vi "solar_excel Worksheet Write (Range).vi"(8 "error in (no error)":errorcluster, 9 "Cells":string[][](array[string]), 10 "Start (1,1 = 'A1')":cluster{"Row":u32, "Column":u32}, 11 "Excel Worksheet in":T1) -> (0 "error out":errorcluster, 3 "Excel Worksheet out":T1)   [LabVIEW 2018]
doc: "This writes <b>Cells</b> to a Worksheet specified by the <b>Start</b> cell range."
uses:
  solar_excel_ctl Worksheet.ctl
  solar_excel_ctl TSV.ctl
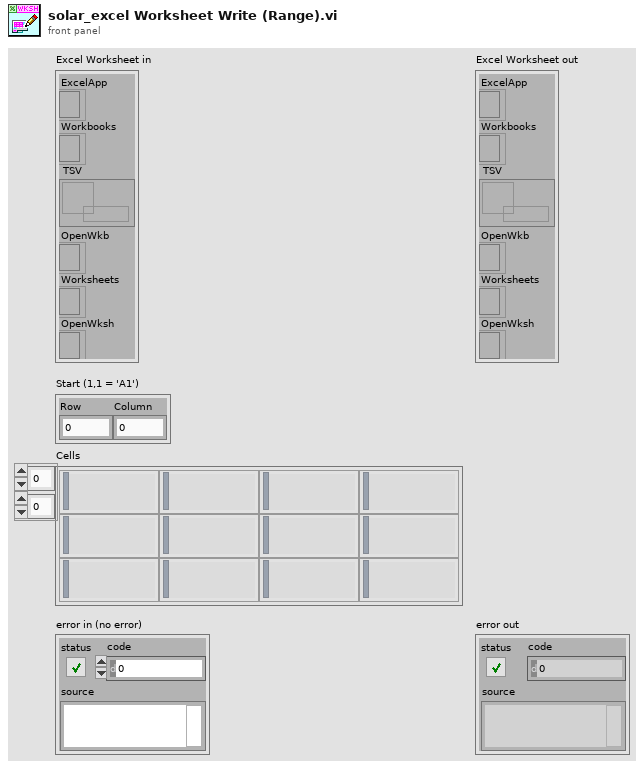
[diagram p1: front panel]
types:
  T1 = typedef "solar_excel_ctl Worksheet.ctl" = cluster{"ExcelApp":refnum<k7>, "Workbooks":refnum<k7>, "TSV":refnum<queue>, "OpenWkb":refnum<k7>, "Worksheets":refnum<k7>, "OpenWksh":refnum<k7>}
  T2 = typedef "solar_excel_ctl TSV.ctl" = cluster{"Path":path, "Dirty":bool, "ActiveSheet":u8, "Worksheets":string[], "Worksheet Cells":cluster{"Cells":string[][]}[]}
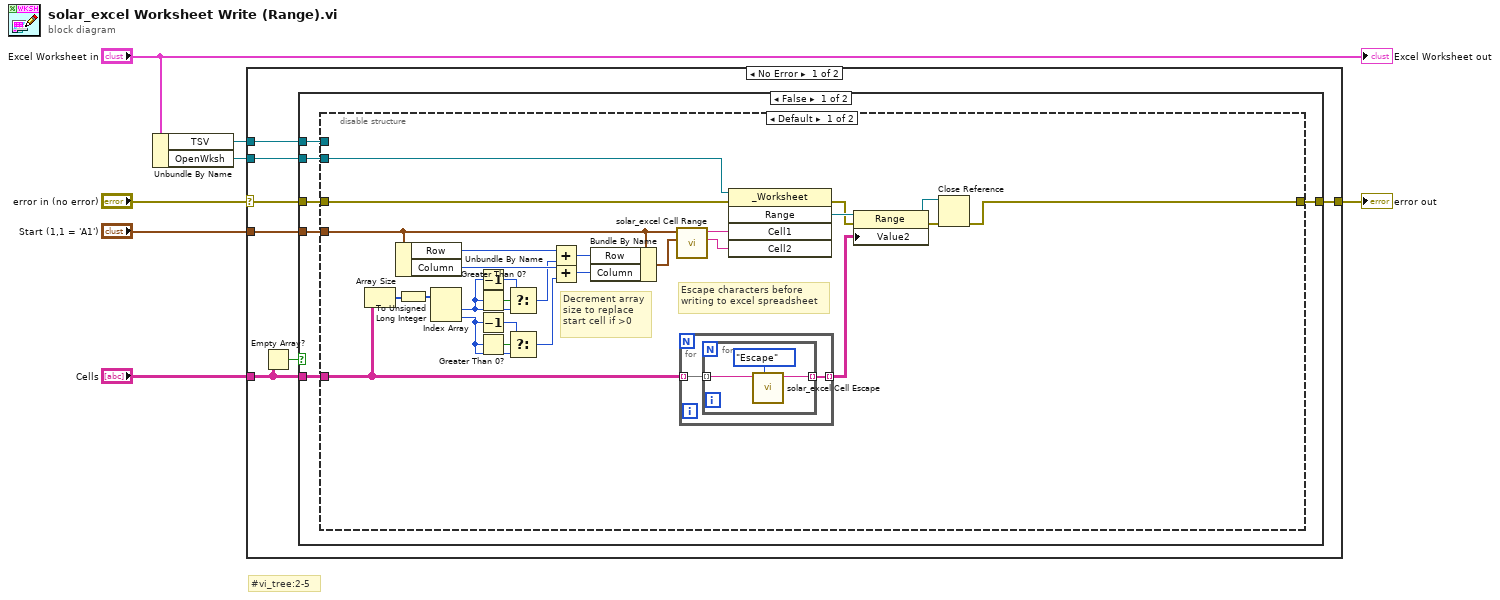
[diagram p0: block diagram]
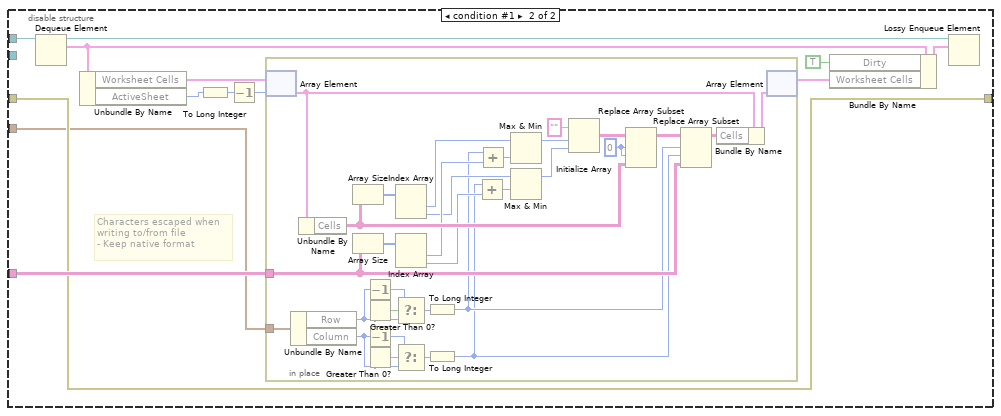
[diagram p2: hidden frame]
diagram:
  # "#vi_tree:2-5"
  n1 = Unbundle By Name("Excel Worksheet in") -> ("TSV"=w1:refnum<queue>, "OpenWksh"=w5:refnum<k7>)
  n2 = case shown="No Error" "error in (no error)" {
    selector: "error in (no error)" -> [w14 w97]
    tunnel: [w12 w97] -> w7
    tunnel: w5 -> [w13 _]
    tunnel: "Start (1,1 = 'A1')" -> [w11 _]
    tunnel: "Cells" -> [w10 _]
    tunnel: w1 -> [w8 _]
    frame No Error {
      n3 = Empty Array?(array=w10) -> (empty?=w9:bool)
      n4 = case shown="False" w9 {
        tunnel: w14 -> [w20 w96]
        tunnel: w13 -> [w19 _]
        tunnel: [w18 w96] -> w12
        tunnel: w10 -> [w17 _]
        tunnel: w11 -> [w16 _]
        tunnel: w8 -> [w15 _]
        frame False {
          n5 = disable-structure shown="Default" {
            disable-tunnel: w20 -> [w47 w54]
            disable-tunnel: w19 -> [w46 _]
            disable-tunnel: [w39 w54] -> w18
            disable-tunnel: w17 -> [w22 w55]
            disable-tunnel: w16 -> [w38 w53]
            disable-tunnel: w15 -> [_ w65]
            frame condition #0 (active) {
              # "Escape characters before\nwriting to excel spreadsheet"
              # "Decrement array\nsize to replace\nstart cell if >0"
              n6 = Array Size(array=w22) -> (size(s)=w36:i32[])
              n7 = Unbundle By Name(w38) -> ("Row"=w35:u32, "Column"=w32:u32)
              n8 = To Unsigned Long Integer(number=w36) -> (unsigned 32bit integer=w33:u32[])
              n9 = Index Array(array=w33) -> (element #1=w24:u32, element #2=w29:u32)  [unwired: 2 in]
              n10 = Decrement(x=w24) -> (x-1=w26:u32)
              n11 = Greater Than 0?(x=w24) -> (x > 0?=w25:bool)
              n12 = Decrement(x=w29) -> (x-1=w28:u32)
              n13 = Greater Than 0?(x=w29) -> (x > 0?=w30:bool)
              n14 = Select(t=w26, s=w25, f=w24) -> (s? t:f=w23:u32)
              n15 = Select(t=w28, s=w30, f=w29) -> (s? t:f=w27:u32)
              n16 = Add(x=w35, y=w23) -> (x+y=w34:u32)
              n17 = Add(x=w32, y=w27) -> (x+y=w31:u32)
              n18 = Bundle By Name(cluster=w38, "Row"=w34, "Column"=w31) -> (w37:cluster{"Row":u32, "Column":u32})
              n19 = call "solar_excel Cell Range.vi"("End (1,1 = 'A1')"=w37, "Start (1,1 = 'A1')"=w38) -> ("End Cell"=w40:string, "Start Cell"=w41:string)  [unwired: 7 in, 1 out]
              n20 = for {
                tunnel: w22 -> [w49] mode=indexing
                tunnel: [w48] -> w21 mode=indexing
                n21 = for {
                  tunnel: w49 -> [w52] mode=indexing
                  tunnel: [w50] -> w48 mode=indexing
                  n22 = call "solar_excel Cell Escape.vi"("Action (Escape)"=enum8{"Escape", "Unescape"}."Escape", "String in"=w52) -> ("String out"=w50:string)  [unwired: 9 in]
                }
              }
              n23 = invoke class="_Worksheet" method="Range"(reference=w46, error in=w47, "Cell1"=w41, "Cell2"=w40) -> (error out=w44:errorcluster, "Range"=w45:refnum<k7>)  [unwired: 1 in, 3 out]
              n24 = property class="Range"(reference=w45, error in=w44, "Value2"=w21) -> (reference out=w42:refnum<k7>, error out=w43:errorcluster)
              n25 = Close Reference(reference=w42, error in (no error)=w43) -> (error out=w39:errorcluster)
            }
            frame condition #1 {
              # "Characters escaped when\nwriting to/from file\n- Keep native format"
              n26 = Dequeue Element(queue=w65) -> (queue out=w64:refnum<queue>, element=w63:T2)  [unwired: 2 in, 2 out]
              n27 = Unbundle By Name(w63) -> ("Worksheet Cells"=w62:cluster{"Cells":string[][]}[], "ActiveSheet"=w61:u8)
              n28 = To Long Integer(number=w61) -> (32bit integer=w60:i32)
              n29 = Decrement(x=w60) -> (x-1=w59:i32)
              n30 = in-place {
                in-place-border: w55 -> [w91]
                in-place-border: w53 -> [w90]
                w77 = 0 ("disabled index (col)")
                n31 = in-place-array #1(w62, w59) -> (w95:cluster{"Cells":string[][]})
                n32 = Unbundle By Name(w90) -> ("Row"=w73:u32, "Column"=w70:u32)
                n33 = Unbundle By Name(w95) -> ("Cells"=w92:string[][])
                n34 = Array Size(array=w92) -> (size(s)=w89:i32[])
                n35 = Array Size(array=w91) -> (size(s)=w88:i32[])
                n36 = Decrement(x=w73) -> (x-1=w74:u32)
                n37 = Greater Than 0?(x=w73) -> (x > 0?=w75:bool)
                n38 = Decrement(x=w70) -> (x-1=w72:u32)
                n39 = Greater Than 0?(x=w70) -> (x > 0?=w71:bool)
                n40 = Index Array(array=w89) -> (element #1=w82:i32, element #2=w80:i32)  [unwired: 2 in]
                n41 = Index Array(array=w88) -> (element #1=w81:i32, element #2=w79:i32)  [unwired: 2 in]
                n42 = Select(t=w74, s=w75, f=w73) -> (s? t:f=w69:u32)
                n43 = Select(t=w72, s=w71, f=w70) -> (s? t:f=w68:u32)
                n44 = To Long Integer(number=w69) -> (32bit integer=w67:i32)
                n45 = To Long Integer(number=w68) -> (32bit integer=w66:i32)
                n46 = Add(x=w66, y=w79) -> (x+y=w85:i32)
                n47 = Add(x=w67, y=w81) -> (x+y=w84:i32)
                n48 = Max & Min(x=w82, y=w84) -> (max(x,y)=w86:i32)  [unwired: 1 out]
                n49 = Max & Min(x=w80, y=w85) -> (max(x,y)=w87:i32)  [unwired: 1 out]
                n50 = Initialize Array("", w86, w87) -> (w76:string[][])
                n51 = Replace Array Subset(array=w76, new element=w92, index (row)=w77, index (col)=w77) -> (w78:string[][])
                n52 = Replace Array Subset(array=w78, new element=w91, index (row)=w67, index (col)=w66) -> (w93:string[][])
                n53 = Bundle By Name(cluster=w95, "Cells"=w93) -> (w94:cluster{"Cells":string[][]})
                n54 = in-place-array #1(w94) -> (w57:cluster{"Cells":string[][]}[])  [unwired: 1 out]
              }
              n55 = Bundle By Name(cluster=w63, "Dirty"=TRUE, "Worksheet Cells"=w57) -> (w58:T2)
              n56 = Lossy Enqueue Element(queue=w64, element=w58) -> ()  [unwired: 1 in, 4 out]
            }
          }
        }
        frame True {
          # "Empty array\n-Do nothing"
        }
      }
    }
    frame Error {
    }
  }
  "error out" <- w7
  "Excel Worksheet out" <- "Excel Worksheet in"
